vi "Start.vi"(8 "error in (no error)":errorcluster, 11 "ConsoleOutput in":refnum<class "ConsoleOutput.lvclass">) -> (0 "error out":errorcluster, 3 "ConsoleOutput out":refnum<class "ConsoleOutput.lvclass">)   [LabVIEW 2020, in "ConsoleOutput.lvclass"]
uses:
  ConsoleOutput.lvclass
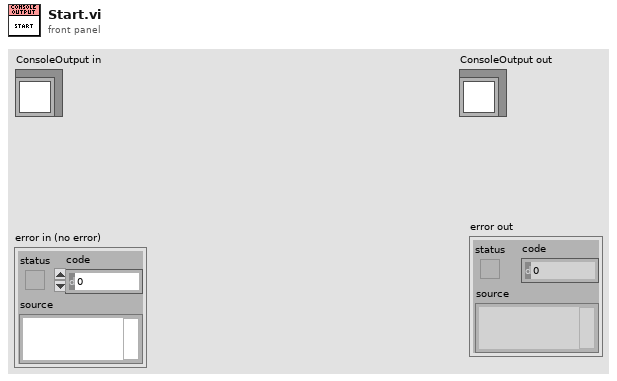
[diagram p1: front panel]
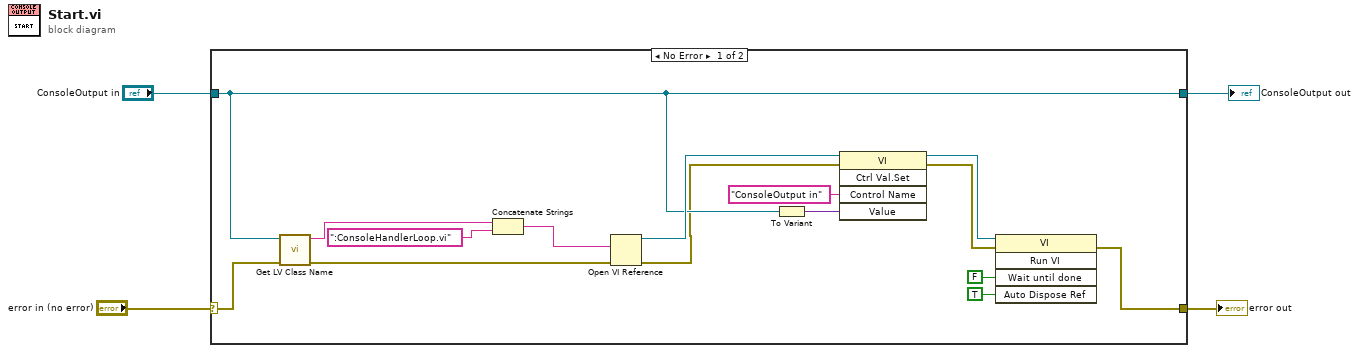
[diagram p0: block diagram]
diagram:
  n1 = case shown="No Error" "error in (no error)" {
    selector: "error in (no error)" -> [w19 w21]
    tunnel: [w5 w21] -> w3
    tunnel: [w10 w20] -> w1
    tunnel: "ConsoleOutput in" -> [w10 w20]
    frame No Error {
      n2 = call <vilib>:"Get LV Class Name.vi"("error in (no error)"=w19, "object"=w10) -> ("error out"=w18:errorcluster, "class name"=w17:string)  [unwired: 8 in]
      n3 = Concatenate Strings(w17, ":ConsoleHandlerLoop.vi" ("string")) -> (w15:string)
      n4 = Open VI Reference(vi path=w15, error in (no error)=w18) -> (vi reference=w11:refnum<vi>, error out=w6:errorcluster)  [unwired: 4 in]
      n5 = To Variant(anything=w10) -> (Variant=w8:variant)
      n6 = invoke class="VI" method="Ctrl Val.Set"(reference=w11, error in=w6, "Control Name"="ConsoleOutput in", "Value"=w8) -> (reference out=w7:refnum<vi>, error out=w12:errorcluster)  [unwired: 1 in, 3 out]
      n7 = invoke class="VI" method="Run VI"(reference=w7, error in=w12, "Wait until done"=FALSE ("Wait Until Done"), "Auto Dispose Ref"=TRUE ("Auto Dispose Reference")) -> (error out=w5:errorcluster)  [unwired: 1 in, 4 out]
    }
    frame Error {
    }
  }
  "error out" <- w3
  "ConsoleOutput out" <- w1
